vi "Log error2.vi"(8 "error in (no error)":errorcluster, 11 "Channel in":refnum<class "Channel.lvclass">) -> (0 "error out":errorcluster, 3 "Channel out":refnum<class "Channel.lvclass">)   [LabVIEW 2018, in "Channel.lvclass"]
uses:
  Channel.lvclass
  Channel.lvclass/Channel.ctl
  Error log/Error log.lvclass
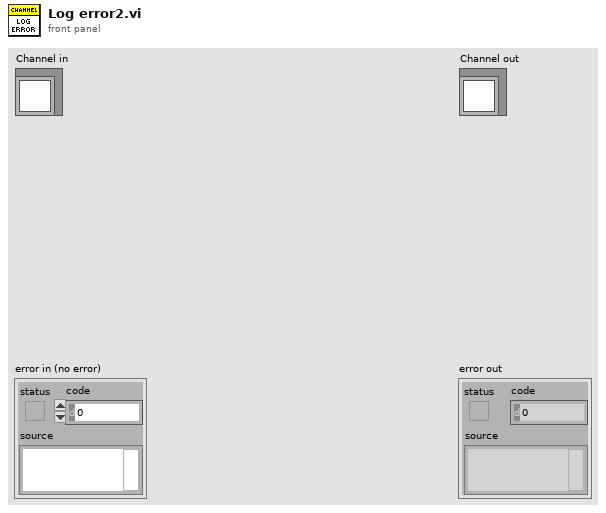
[diagram p1: front panel]
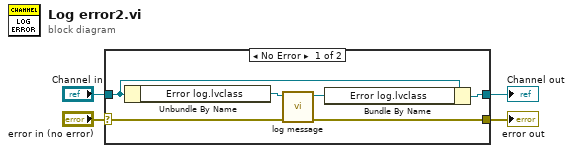
[diagram p0: block diagram]
diagram:
  n1 = case shown="No Error" "error in (no error)" {
    selector: "error in (no error)" -> [w8 w12]
    tunnel: [w7 w12] -> w3
    tunnel: [w9 w11] -> w1
    tunnel: "Channel in" -> [w10 w11]
    frame No Error {
      n2 = Unbundle By Name(w10) -> ("Error log.lvclass"=w5:refnum<class "Error log.lvclass">)
      n3 = call-dynamic "log message.vi"("error in (no error)"=w8, "Error log in"=w5) -> ("error out"=w7:errorcluster, "Error log out"=w6:refnum<class "Error log.lvclass">)  [unwired: 8 in]
      n4 = Bundle By Name(cluster=w10, "Error log.lvclass"=w6) -> (w9:refnum<class "Channel.lvclass">)
    }
    frame Error {
    }
  }
  "error out" <- w3
  "Channel out" <- w1
